vi "KM_appendline -- freq sweep.vi"(1 "freq":dbl[](array[numeric]), 2 "Vout(V)":cdb[](array[numeric]), 5 "header":string="frequency(Hz) Vx(V) Vy(V)", 7 "Save frequency scan":path=path "C:/data/Ultrasound/birdcage/Hg1201/Test", 8 "read/write control":T1, 9 "name or relative path":string) -> ()   [LabVIEW 2021]
uses:
  KM_file -- read-write control.ctl
  file -- read-write control.ctl
  <vilib>/Utility/libraryn.llb/Check if File or Folder Exists.vi
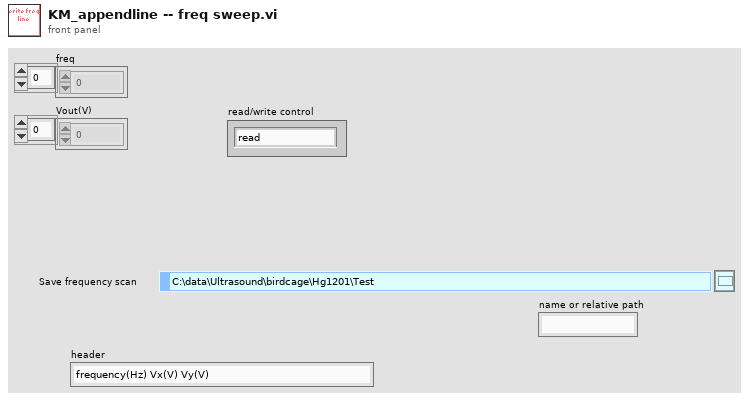
[diagram p1: front panel]
types:
  T1 = typedef "KM_file -- read-write control.ctl" = enum16{"read", "write all", "append one line"}
  T2 = typedef "file -- read-write control.ctl" = enum16{"read", "write all", "append one line"}
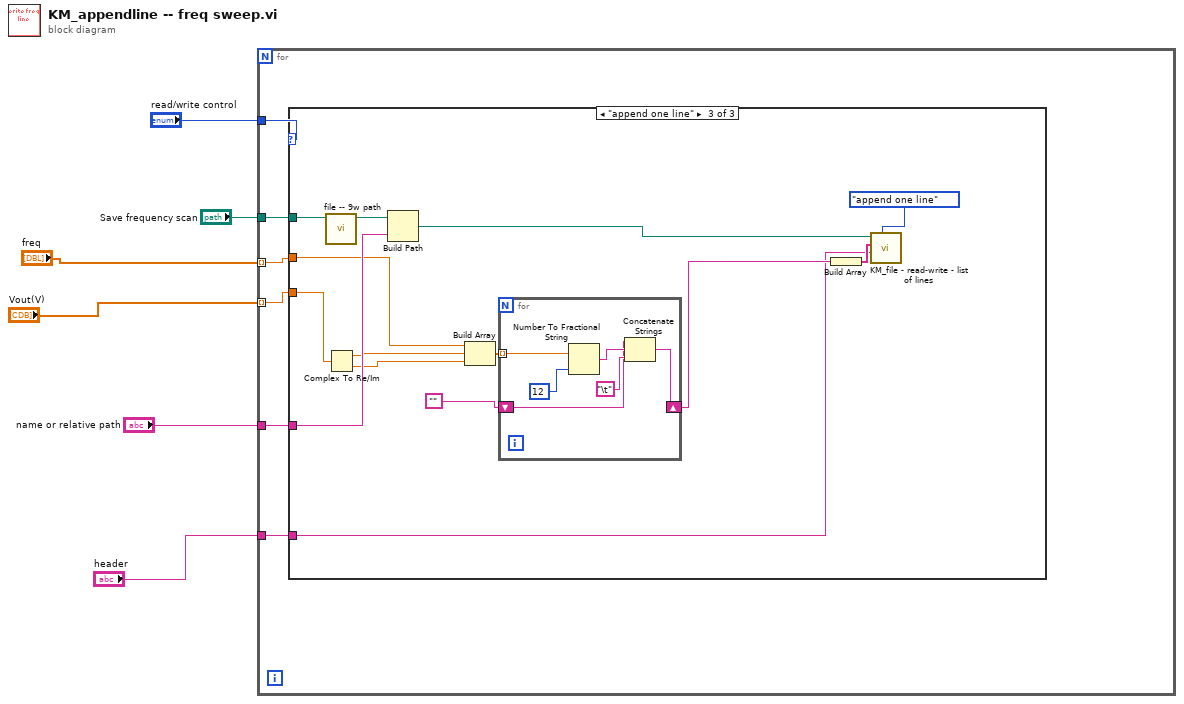
[diagram p0: block diagram]
diagram:
  n1 = for {
    tunnel: "read/write control" -> [w12]
    tunnel: "Save frequency scan" -> [w11]
    tunnel: "name or relative path" -> [w10]
    tunnel: "freq" -> [w9] mode=indexing
    tunnel: "Vout(V)" -> [w8] mode=indexing
    tunnel: "header" -> [w7]
    n2 = case shown="\"append one line\"" w12 {
      tunnel: w11 -> [_ _ w26]
      tunnel: w10 -> [_ _ w24]
      tunnel: w8 -> [_ _ w16]
      tunnel: w9 -> [_ _ w17]
      tunnel: w7 -> [_ _ w13]
      frame "read", Default {
      }
      frame "write all" {
      }
      frame "append one line" {
        n3 = call "file -- 9w path.vi"("sweep folder"=w26) -> ("9w path"=w25:path)  [unwired: 10 in]
        n4 = Complex To Re/Im(x + iy=w16) -> (x=w15:dbl, y=w14:dbl)
        n5 = Build Path(base path=w25, name or relative path=w24) -> (appended path=w19:path)
        n6 = Build Array(w17, w15, w14) -> (w23:dbl[])
        n7 = for {
          tunnel: w23 -> [w32] mode=indexing
          shift-right: [w28] -> w21
          shift-left: "" -> [w29]
          n8 = Number To Fractional String(number=w32, precision (6)=i16 12) -> (F-format string=w31:string)  [unwired: 2 in]
          n9 = Concatenate Strings(w29, w31, "\t" ("string")) -> (w28:string)
        }
        n10 = Build Array(w21) -> (w18:string[])
        n11 = call "KM_file - read-write - list of lines.vi"("read/write control"=file_--_read-write_control."append one line", "header"=w13, "list of lines IN"=w18, "file path"=w19) -> ()  [unwired: 6 in, 2 out]
      }
    }
  }
